vi "LEP_RV_IsLaunching.vi"() -> (3 "not in memory":bool)   [LabVIEW 2011]
doc: "Download and execute built VxWorks downloadable module and attach the LabVIEW Embedded debuger."
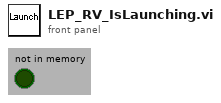
[diagram p1: front panel]
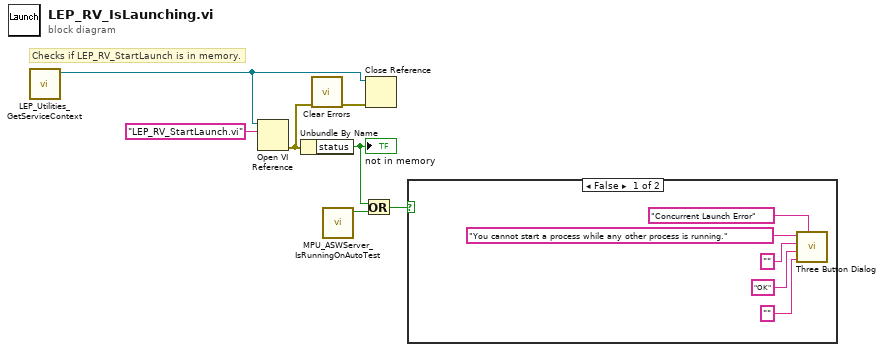
[diagram p0: block diagram]
diagram:
  # "Checks if LEP_RV_StartLaunch is in memory."
  n1 = call <vilib>:"LEP_Utilities_GetServiceContext.vi"() -> ("service context"=w6:refnum<vi>)  [unwired: 1 in, 10 out]
  n2 = Open VI Reference(application reference (local)=w6, vi path="LEP_RV_StartLaunch.vi") -> (error out=w5:errorcluster)  [unwired: 4 in, 1 out]
  n3 = Unbundle By Name(w5) -> ("status"=w3:bool)
  "not in memory" <- w3
  n4 = call <vilib>:"Clear Errors.vi"("error in (no error)"=w5) -> ("error out"=w4:errorcluster)  [unwired: 6 in]
  n5 = call <vilib>:"MPU_ASWServer_IsRunningOnAutoTest.vi"() -> ("running in autotest?"=w2:bool)  [unwired: 1 in, 10 out]
  n6 = Or(x=w3, y=w2) -> (x .or. y?=w1:bool)
  n7 = Close Reference(reference=w6, error in (no error)=w4) -> ()  [unwired: 1 out]
  n8 = case shown="False" w1 {
    frame False {
      n9 = call <vilib>:"Three Button Dialog.vi"("Window Title (\"\")"="Concurrent Launch Error" ("Window Title (\"\")"), "Right Button Text (\"Cancel\")"="" ("Right Button Text (\"Cancel\")"), "Center Button Text (\"No\")"="OK" ("Center Button Text (\"No\")"), "Left Button Text (\"Yes\")"="" ("Left Button Text (\"Yes\")"), "message"="You cannot start a process while any other process is running.") -> ()  [unwired: 6 in, 1 out]
    }
    frame True {
    }
  }
